vi "Lift.vi"(11 "output cluster":T1) -> ()   [LabVIEW 2016]
uses:
  Joystick/ControlsToCommands.ctl
  References/Refnums.vi
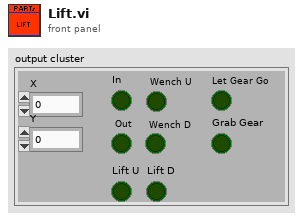
[diagram p1: front panel]
types:
  T1 = typedef "ControlsToCommands.ctl" = cluster{"X":dbl, "Y":dbl, "In":bool, " Out":bool, "Lift U":bool, " Wench U":bool, " Wench D":bool, "Lift D":bool, "Let Gear Go":bool, "Grab Gear":bool}
  T2 = typedef "WPI_MotorControlDeviceRef.ctl" = cluster{"DeviceStatus":errorcluster, "Type":T3, "PWM":cluster{"PWM Channel":T4, "DeadBand":T5}, "CAN":cluster{"Device Number":u8, "SetOutput VI Ref":variant, "GetOutput VI Ref":variant, "Enable VI Ref":variant, "Disable VI Ref":variant, "Data":variant}, "Invert":bool}
  T3 = typedef "WPI_MotorControlType.ctl" = enum16{"PWM", "CAN"}
  T4 = typedef "FPGA_DIOPWMChannel.ctl" = enum8{"PWM 0", "PWM 1", "PWM 2", "PWM 3", "PWM 4", "PWM 5", "PWM 6", "PWM 7", "PWM 8", "PWM 9", "PWM MXP 0", "PWM MXP 1", "PWM MXP 2", "PWM MXP 3", "PWM MXP 4", "PWM MXP 5", "PWM MXP 6", "PWM MXP 7", "PWM MXP 8", "PWM MXP 9", "Invalid"}
  T5 = typedef "WPI_PWMDeadband.ctl" = cluster{"Name":string, "maxPositivePwm":i32, "minPositivePwm":i32, "centerPwm":i32, "maxNegativePwm":i32, "minNegativePwm":i32, "angularRange":u16}
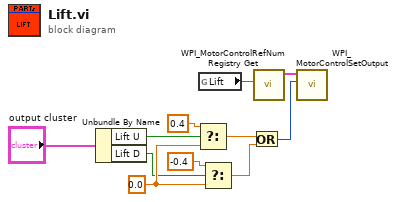
[diagram p0: block diagram]
diagram:
  w5 = 0.0 ("f")
  n1 = Unbundle By Name("output cluster") -> ("Lift U"=w3:bool, "Lift D"=w4:bool)
  n2 = Select(t=0.4, s=w3, f=w5) -> (s? t:f=w8:dbl)
  n3 = global read "Refnums.vi" "Lift"() -> (w11:string)
  n4 = Select(t=-0.4, s=w4, f=w5) -> (s? t:f=w9:dbl)
  n5 = Or(x=w8, y=w9) -> (x .or. y?=w10:i32)
  n6 = call <vilib>:"WPI_MotorControlRefNum Registry Get.vi"("refnum name"=w11) -> ("MotorControlDevRef"=w1:T2)  [unwired: 9 in, 1 out]
  n7 = call <vilib>:"WPI_MotorControlSetOutput.vi"("Output"=w10, "MotorControlDevRef"=w1) -> ()  [unwired: 7 in, 3 out]
